vi "Transform3d_Create_Pose3dPose3d.vi"(9 "last Pose3d":T1={"Translation3d"={"X"=0.0, "Y"=0.0, "Z"=0.0}, "Rotation3d"={"Q_quaternion"={"R"=1.0, "V"=[0.0, 0.0, 0.0]}}} {"Translation3d"."Z" format="%14.3f"; "Translation3d"."Y" format="%14.3f"; "Translation3d"."X" format="%14.3f"}, 11 "initial Pose3d":T1={"Translation3d"={"X"=0.0, "Y"=0.0, "Z"=0.0}, "Rotation3d"={"Q_quaternion"={"R"=1.0, "V"=[0.0, 0.0, 0.0]}}} {"Translation3d"."Z" format="%14.3f"; "Translation3d"."Y" format="%14.3f"; "Translation3d"."X" format="%14.3f"}) -> (3 "Transform3d":T5={"TRANSLATION3D"={"X"=0.0, "Y"=0.0, "Z"=0.0}, "ROTATION3D"={"Q_quaternion"={"R"=1.0, "V"=[0.0, 0.0, 0.0]}}, "XF"=FALSE} {"TRANSLATION3D"."Z" format="%14.3f"; "TRANSLATION3D"."Y" format="%14.3f"; "TRANSLATION3D"."X" format="%14.3f"})   [LabVIEW 2019, in "Trajectory_Library.lvlib"]
doc: "Constructs the transform that maps the initial pose to the final pose.\n\nParameters:\n - initial pose3d -- The initial pose for the transformation.\n - last pose3d -- The final pose for the transformation.\n\nReturns:\n - Transform 3d -- The TRANSFORM3d data structure"
uses:
  Trajectory_Library.lvlib
  TypeDef/TRANSLATION3D.ctl
  TypeDef/QUATERNION.ctl
  TypeDef/ROTATION3D.ctl
  TypeDef/POSE3D.ctl
  TypeDef/TRANSFORM3D.ctl
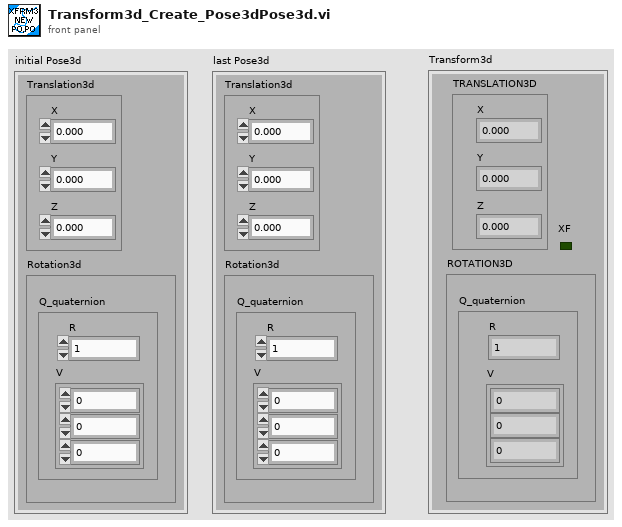
[diagram p1: front panel]
types:
  T1 = typedef "Trajectory_Library.lvlib/POSE3D.ctl" = cluster{"Translation3d":T2, "Rotation3d":T3}
  T2 = typedef "Trajectory_Library.lvlib/TRANSLATION3D.ctl" = cluster{"X":dbl, "Y":dbl, "Z":dbl}
  T3 = typedef "Trajectory_Library.lvlib/ROTATION3D.ctl" = cluster{"Q_quaternion":T4}
  T4 = typedef "Trajectory_Library.lvlib/QUATERNION.ctl" = cluster{"R":dbl, "V":dbl[]}
  T5 = typedef "Trajectory_Library.lvlib/TRANSFORM3D.ctl" = cluster{"TRANSLATION3D":T2, "ROTATION3D":T3, "XF":bool}
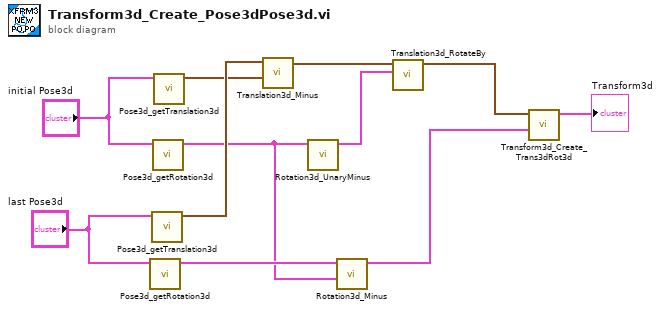
[diagram p0: block diagram]
diagram:
  n1 = call "Pose3d_getRotation3d.vi"("in Pose3d"="last Pose3d") -> ("out Rotation3d"=w3:T3)  [unwired: 10 in]
  n2 = call "Pose3d_getTranslation3d.vi"("in Pose3d"="last Pose3d") -> ("out Translation3d"=w8:T2)  [unwired: 10 in]
  n3 = call "Pose3d_getRotation3d.vi"("in Pose3d"="initial Pose3d") -> ("out Rotation3d"=w2:T3)  [unwired: 10 in]
  n4 = call "Pose3d_getTranslation3d.vi"("in Pose3d"="initial Pose3d") -> ("out Translation3d"=w7:T2)  [unwired: 10 in]
  n5 = call "Translation3d_Minus.vi"("other Translation3d"=w7, "In Translation3d"=w8) -> ("Out Translation3d"=w6:T2)  [unwired: 9 in]
  n6 = call "Rotation3d_UnaryMinus.vi"("in Rotation3d"=w2) -> ("out Rotation3d"=w5:T3)  [unwired: 10 in]
  n7 = call "Rotation3d_Minus.vi"("other Rotation3d"=w2, "in Rotation3d"=w3) -> ("out Rotation3d"=w1:T3)  [unwired: 9 in]
  n8 = call "Translation3d_RotateBy.vi"("other Rot3d"=w5, "in Translation3D"=w6) -> ("out Translation3d"=w4:T2)  [unwired: 9 in]
  n9 = call "Transform3d_Create_Trans3dRot3d.vi"("Rotation3d"=w1, "Translation3d"=w4) -> ("Transform3d"=→"Transform3d":T5)  [unwired: 9 in]
